vi "Create ChildClass.vi"(5 "ChildClass in":refnum<class "ChildClass.lvclass">, 8 "error in (no error)":errorcluster, 10 "String":string, 11 "Numeric":dbl) -> (0 "error out":errorcluster, 3 "ChildClass":refnum<class "ChildClass.lvclass">)   [LabVIEW 2017, in "TestLibrary.lvlib" / "ChildClass.lvclass"]
uses:
  ChildClass.lvclass
  C:/Users/pasca/Projects/Home/labview-composition/Tests/PPL_Inheritance/TestLibrary/ParentClass/ParentClass.lvclass
  ChildClass.lvclass/ChildClass.ctl
  ParentClass/ParentClass.lvclass
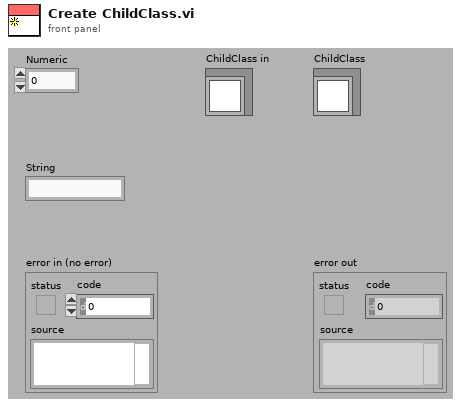
[diagram p1: front panel]
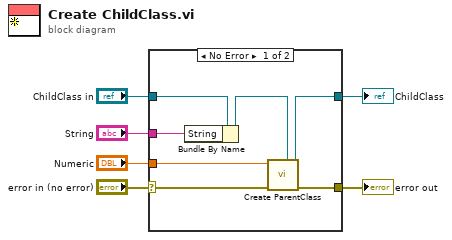
[diagram p0: block diagram]
diagram:
  n1 = case shown="No Error" "error in (no error)" {
    selector: "error in (no error)" -> [w8 w15]
    tunnel: [w7 w15] -> w5
    tunnel: [w9 w14] -> w3
    tunnel: "ChildClass in" -> [w13 w14]
    tunnel: "String" -> [w12 _]
    tunnel: "Numeric" -> [w11 _]
    frame No Error {
      n2 = Bundle By Name(cluster=w13, "String"=w12) -> (w10:refnum<class "ChildClass.lvclass">)
      n3 = call "Create ParentClass.vi"("ParentClass in"=w10, "error in (no error)"=w8, "Numeric"=w11) -> ("error out"=w7:errorcluster, "ParentClass"=w9:refnum<class "ChildClass.lvclass">)  [unwired: 7 in]
    }
    frame Error {
    }
  }
  "error out" <- w5
  "ChildClass" <- w3
